vi "read command.vi"(8 "error in (no error)":errorcluster, 11 "Request in":refnum<class "Request.lvclass">) -> (0 "error out":errorcluster, 2 "command":T1, 3 "Request out":refnum<class "Request.lvclass">)   [LabVIEW 2018, in "Request.lvclass"]
uses:
  Request.lvclass
  Request.lvclass/Request.ctl
  Command/Command.lvclass/Command.ctl
  Command/Command.lvclass
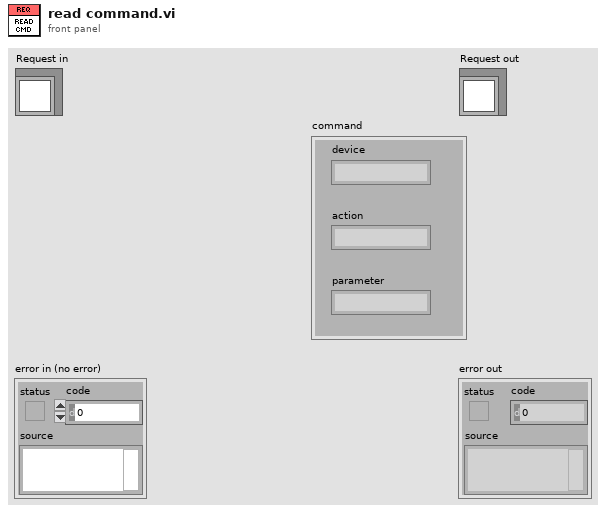
[diagram p1: front panel]
types:
  T1 = cluster{"device":string, "action":string, "parameter":string}
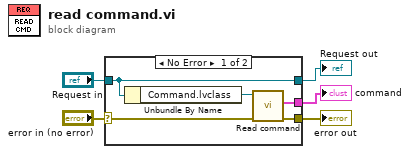
[diagram p0: block diagram]
diagram:
  n1 = case shown="No Error" "error in (no error)" {
    selector: "error in (no error)" -> [w8 w12]
    tunnel: [w7 w12] -> w4
    tunnel: [w10 w11] -> w2
    tunnel: "Request in" -> [w10 w11]
    tunnel: [w6 _] -> w1
    frame No Error {
      n2 = Unbundle By Name(w10) -> ("Command.lvclass"=w9:refnum<class "Command.lvclass">)
      n3 = call "Read command.vi"("error in (no error)"=w8, "Command in"=w9) -> ("error out"=w7:errorcluster, "command"=w6:T1)  [unwired: 7 in, 1 out]
    }
    frame Error {
    }
  }
  "error out" <- w4
  "Request out" <- w2
  "command" <- w1
